vi "Main.vi"() -> ()   [LabVIEW 2016]
doc: "The myRIO Project template acquires acceleration data from the onboard accelerometer and displays the changes of acceleration values in a waveform chart."
uses:
  <vilib>/myRIO/Instrument Drivers/Onboard IO/PWM/typedefs/PWM Reference.ctl
  <vilib>/myRIO/Common/Instrument Driver Framework/Utilities/typedefs/myRIO Generic Hardware Reference.ctl
  <vilib>/myRIO/Common/Instrument Driver Framework/Utilities/typedefs/Hardware Version Enum.ctl
  <vilib>/myRIO/Common/Instrument Driver Framework/Utilities/typedefs/myRIO v1.0 Reference.ctl
  <vilib>/myRIO/Common/Instrument Driver Framework/Utilities/typedefs/Generic FPGA Reference.ctl
  <vilib>/myRIO/Common/Instrument Driver Framework/myRIO v1.0/PWM/typedefs/PWM Channels Enum.ctl
  <vilib>/myRIO/Instrument Drivers/Onboard IO/PWM/typedefs/PWM Configuration.ctl
  <vilib>/userdefined/High Color/nirio_resource_hc.ctl
  <vilib>/myRIO/Common/Instrument Driver Framework/myRIO v1.0/PWM/vis/myRIO v1.1 Open PWM.vi
  <vilib>/myRIO/Common/Instrument Driver Framework/Utilities/vis/Validate Channels.vi
  <vilib>/myRIO/Common/Instrument Driver Framework/myRIO v1.0/PWM/vis/myRIO v1.0 Reserve PWM.vi
  <vilib>/myRIO/Common/Instrument Driver Framework/myRIO v1.0/UART/vis/myRIO v1.0 Close UART.vi
  <vilib>/myRIO/Common/Instrument Driver Framework/myRIO v1.0/PWM/vis/myRIO v1.0 Build MUX Configuration PWM.vi
  <vilib>/myRIO/Common/Instrument Driver Framework/myRIO v1.0/Resource Manager/vis/myRIO v1.0 Reserve Channel List.vi
  <vilib>/myRIO/Common/Instrument Driver Framework/myRIO v1.0/Resource Manager/vis/myRIO v1.0 Create Configuration List.vi
  <vilib>/myRIO/Common/Instrument Driver Framework/myRIO v1.0/Resource Manager/vis/myRIO v1.0 Reserve Channel.vi
  <vilib>/myRIO/Common/Instrument Driver Framework/myRIO v1.0/Resource Manager/vis/myRIO v1.0 Unreserve Channel.vi
  <vilib>/myRIO/Common/Instrument Driver Framework/myRIO v1.0/Resource Manager/vis/myRIO v1.0 Build Mutex Name.vi
  <vilib>/Utility/VariantDataType/GetNumericInfo.vi
  <vilib>/Utility/error.llb/Error Cluster From Error Code.vi
  <vilib>/myRIO/Common/Instrument Driver Framework/myRIO v1.0/myRIO v1.1 Open.vi
  <vilib>/myRIO/Common/Instrument Driver Framework/Utilities/vis/IO Manager.vi
  <vilib>/myRIO/Common/Instrument Driver Framework/Utilities/vis/Configuration Manager.vi
  <vilib>/myRIO/Common/Instrument Driver Framework/myRIO v1.0/Resource Manager/vis/myRIO v1.0 Configure IO.vi
  <vilib>/myRIO/Common/Instrument Driver Framework/myRIO v1.0/myRIO v1.0 Close.vi
  <vilib>/addons/control/pid/pid.llb/PID (DBL).vi
  <vilib>/myRIO/Common/Instrument Driver Framework/myRIO v1.0/PWM/vis/myRIO v1.0 Write PWM.vi
  <vilib>/myRIO/Common/Instrument Driver Framework/Utilities/vis/FPGA Ref Manager.vi
  <vilib>/myRIO/Common/Instrument Driver Framework/myRIO v1.0/myRIO v1.0 Reset FPGA.vi
  <vilib>/myRIO/Common/Instrument Driver Framework/myRIO v1.0/IRQ/vis/myRIO v1.0 IRQ Info FGV.vi
  <vilib>/myRIO/Common/Instrument Driver Framework/myRIO v1.0/IRQ/vis/myRIO v1.0 Timer IRQ Info FGV.vi
  <vilib>/myRIO/Common/Instrument Driver Framework/myRIO v1.0/IRQ/vis/myRIO v1.0 ISR Agent.vi
  <vilib>/myRIO/Instrument Drivers/Onboard IO/PWM/vis/myRIO PWM Open.xnode
  <vilib>/myRIO/Instrument Drivers/Onboard IO/PWM/PWM.lvlib
  <vilib>/myRIO/Instrument Drivers/Utilities/Utilities.lvlib
  <vilib>/addons/control/pid/NI_PID_pid.lvlib
panel:
  out "output array":dbl[](array[numeric])
  in  "Stop Button":bool
  in  "y":dbl(knob) scale=0.0..1.0
  out "pwm motor":dbl
  in  "Frequenz Motor":dbl=200.0
  in  "stop 2":bool
  in  "PID gains":T1={"proportional gain (Kc)"=0.71, "integral time (Ti, min)"=2.0, "derivative time (Td, min)"=0.0015} {"derivative time (Td, min)" format="%.3f"; "integral time (Ti, min)" format="%.3f"; "proportional gain (Kc)" format="%.3f"}
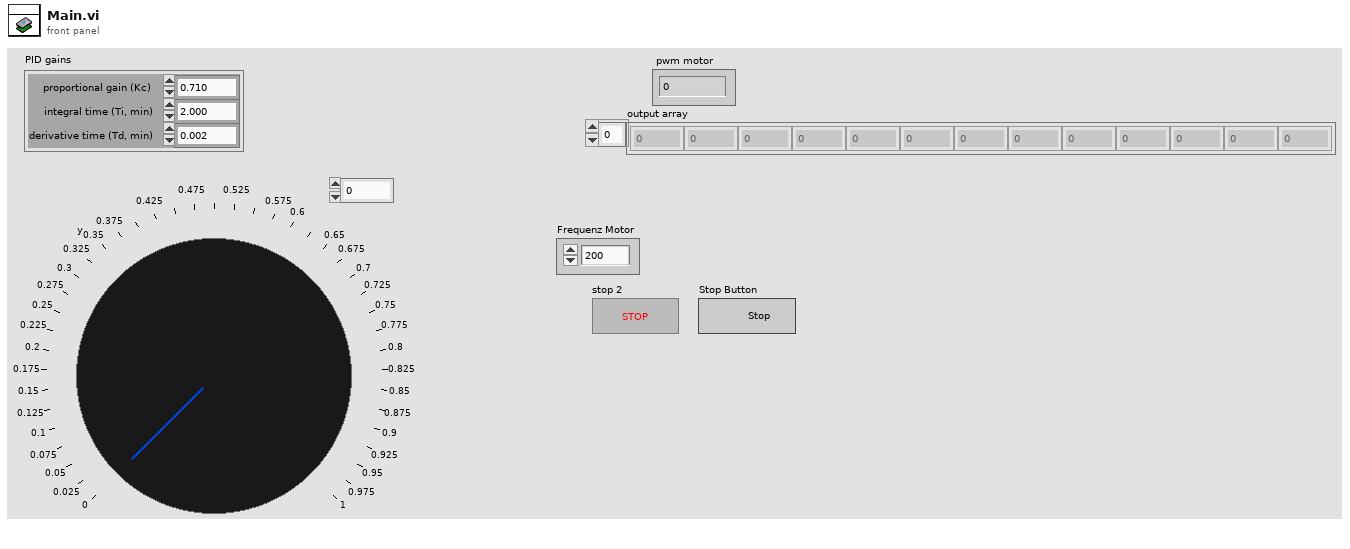
[diagram p1: front panel]
types:
  T1 = cluster{"proportional gain (Kc)":dbl, "integral time (Ti, min)":dbl, "derivative time (Td, min)":dbl}
  T2 = typedef "PWM.lvlib/PWM Reference.ctl" = cluster{"myRIO Reference":T3, "PWM Channels Enum":T7, "PWM Configuration":T8}
  T3 = typedef "myRIO Generic Hardware Reference.ctl" = cluster{"myRIO Model":T4, "myRIO Hardware Reference":T5}
  T4 = typedef "Hardware Version Enum.ctl" = enum16{"Unknown", "myRIO-1900", "myRIO-1950", "roboRIO", "NI ELVIS RIO CM"}
  T5 = typedef "myRIO v1.0 Reference.ctl" = cluster{"Generic FPGA Reference":T6, "Allow multiple opens":bool}
  T6 = typedef "Generic FPGA Reference.ctl" = refnum<k20>
  T7 = typedef "PWM Channels Enum.ctl" = enum16{"Not Connected", "C/PWM0", "C/PWM1", "A/PWM0", "A/PWM1", "A/PWM2", "B/PWM0", "B/PWM1", "B/PWM2", "PWM/PWM0", "PWM/PWM1", "PWM/PWM2", "PWM/PWM3", "PWM/PWM4", "PWM/PWM5", "PWM/PWM6", "PWM/PWM7", "PWM/PWM8", "PWM/PWM9"}
  T8 = typedef "PWM.lvlib/PWM Configuration.ctl" = cluster{"Frequency":dbl, "Duty Cycle":dbl}
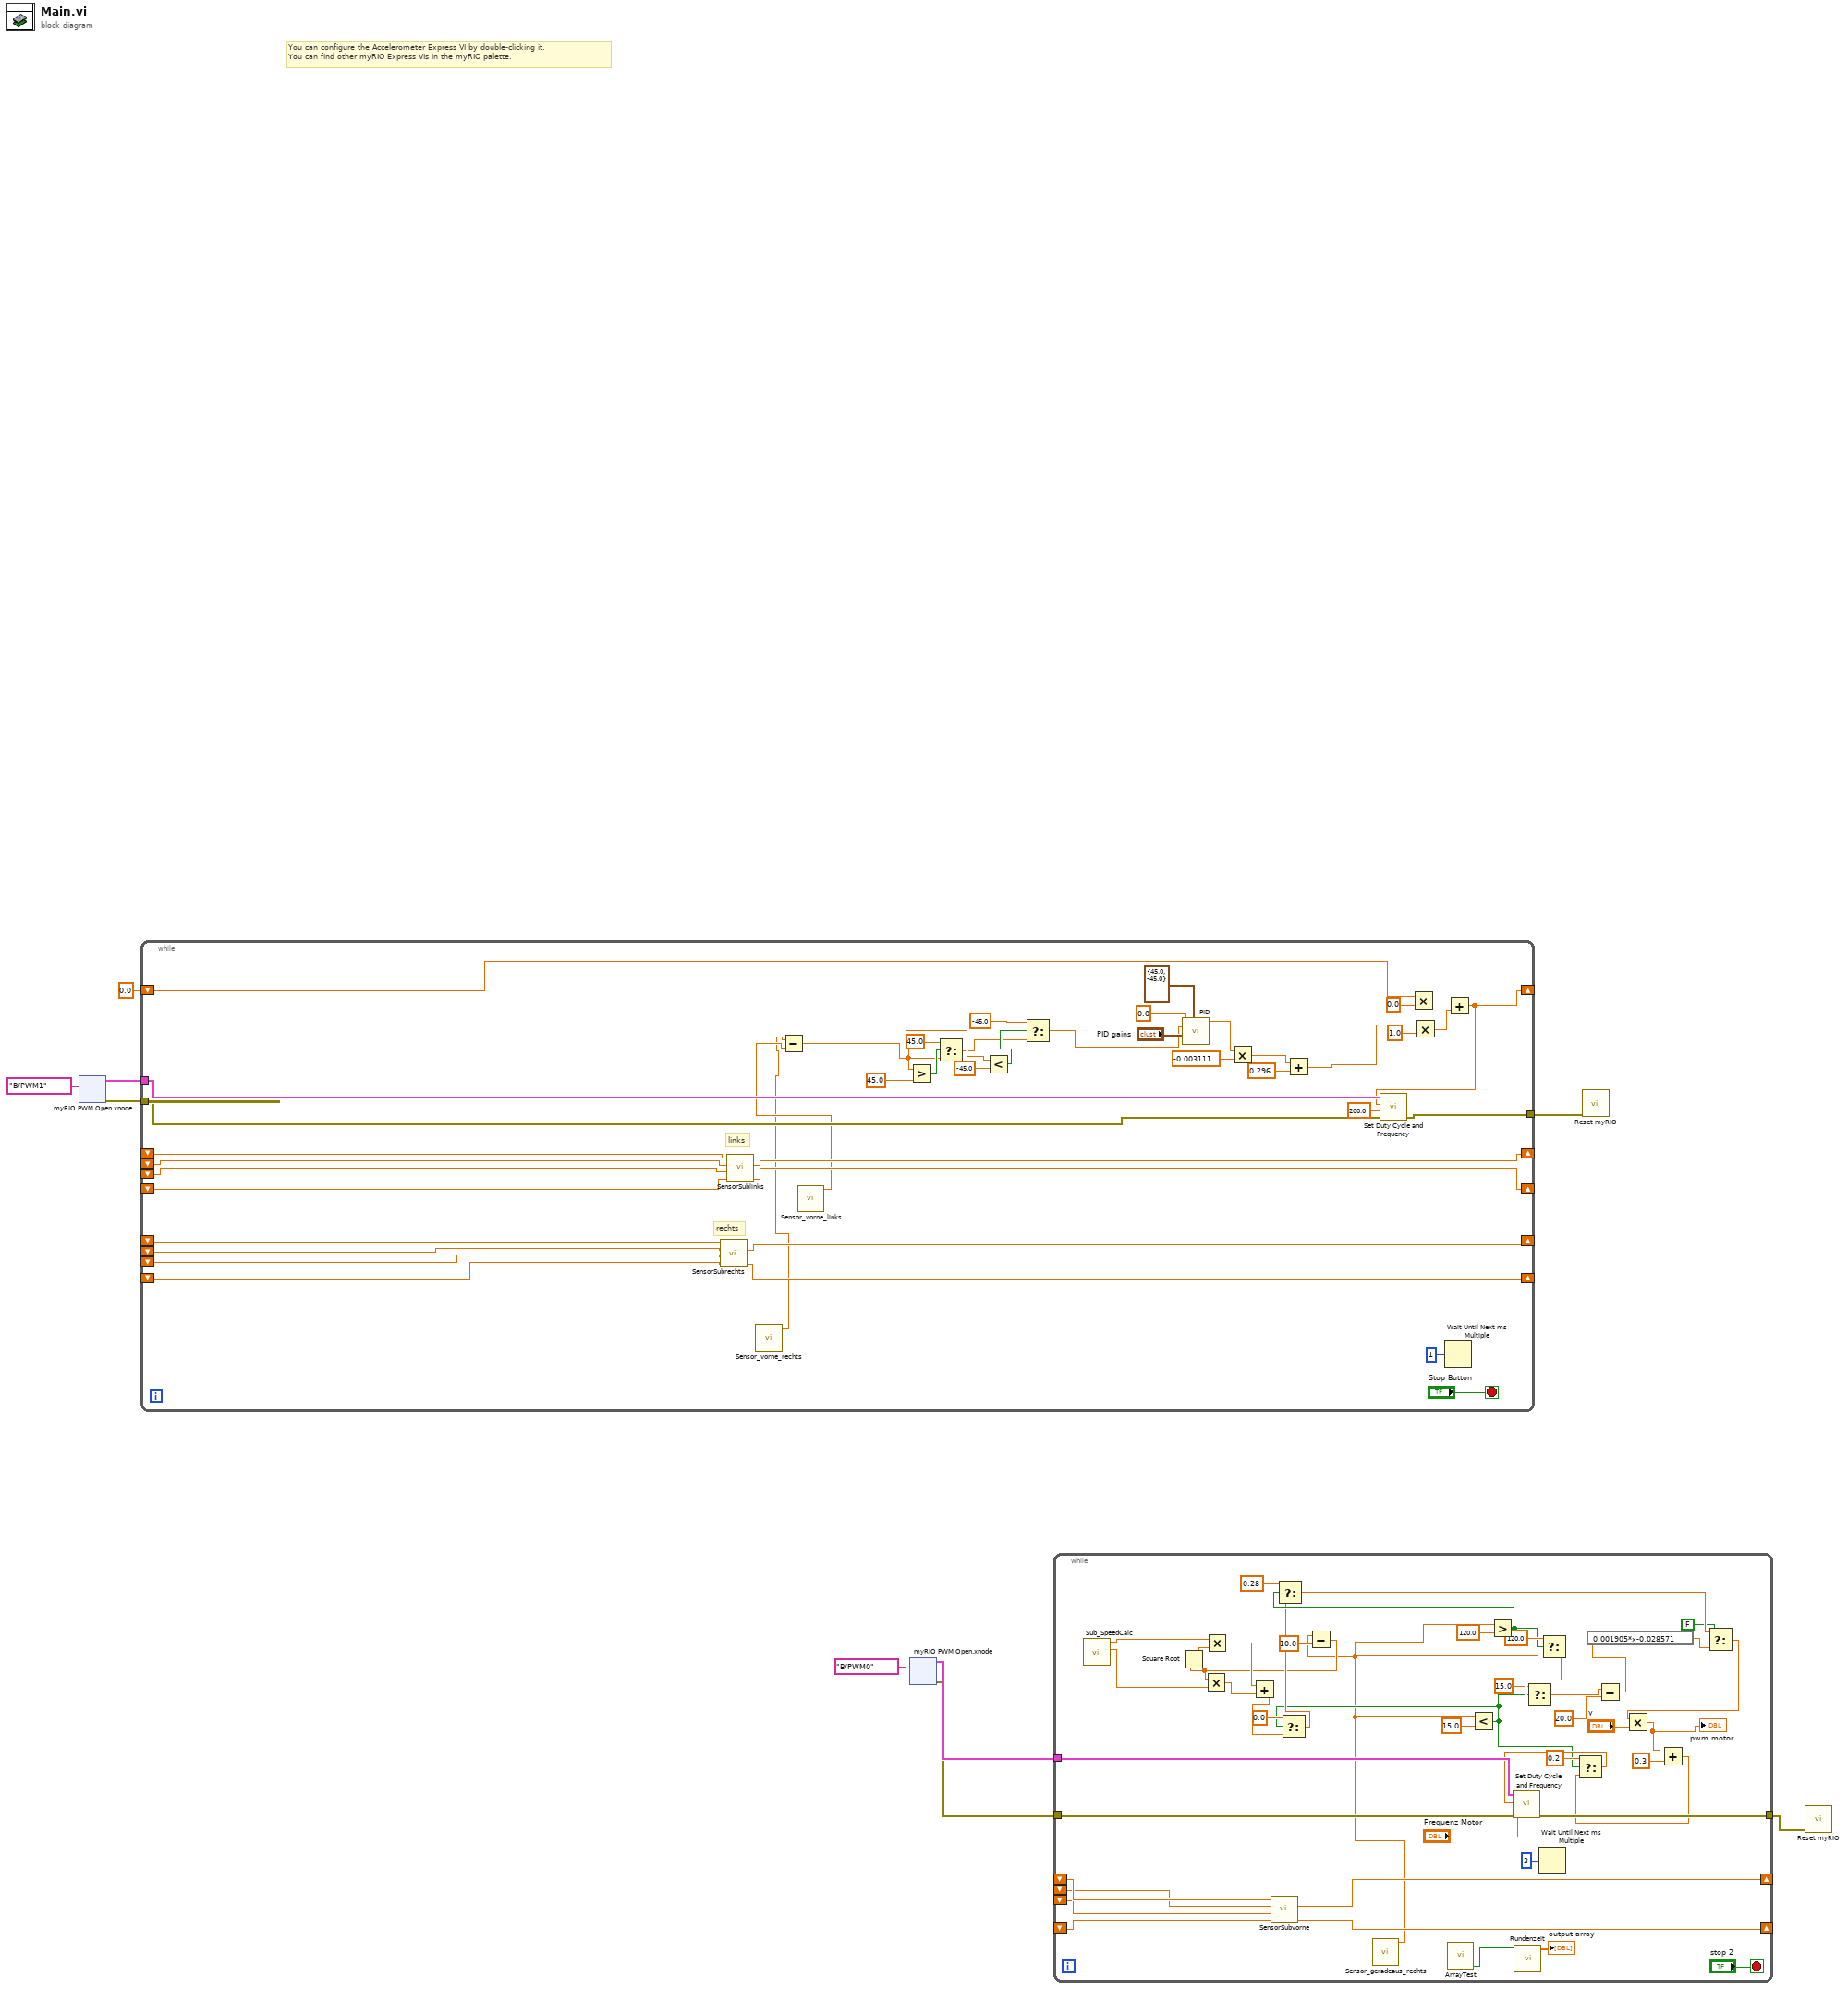
[diagram p0: block diagram]
diagram:
  # "You can configure the Accelerometer Express VI by double-clicking it.\nYou can find other myRIO Express VIs in the myRIO palette."
  n1 = xnode "myRIO PWM Open.xnode"("Channel Name"=tag "B/PWM1") -> ("error out"=w8:errorcluster, "PWM Ref Out"=w7:T2)  [unwired: 2 in]
  n2 = while {
    tunnel: w8 -> [w50]
    tunnel: w7 -> [w52]
    tunnel: [w51] -> w6
    shift-right: [w30] -> _
    shift-left: _ -> [w31]
    shift-right: [w29] -> _
    shift-left: _ -> [w34]
    shift-left: _ -> [w33]
    shift-left: _ -> [w32]
    shift-right: [w42] -> _
    shift-left: 0.0 -> [w45]
    shift-right: [w23] -> _
    shift-left: _ -> [w28]
    shift-left: _ -> [w27]
    shift-left: _ -> [w26]
    shift-right: [w24] -> _
    shift-left: _ -> [w25]
    stop <- "Stop Button" stop-if-true
    # "links"
    # "rechts"
    n3 = call "SensorSubrechts.vi"("Tiefpass in"=w25, "element 3"=w26, "element 2"=w27, "element"=w28) -> ("Tiefpass out"=w24:dbl, "Ausgabe IR"=w23:dbl)  [unwired: 5 in, 1 out]
    n4 = call "SensorSublinks.vi"("Tiefpass in"=w31, "element 3"=w32, "element 2"=w33, "element"=w34) -> ("Tiefpass out"=w30:dbl, "Ausgabe IR"=w29:dbl)  [unwired: 5 in, 1 out]
    n5 = call "Sensor_vorne_rechts.vi"() -> ("Abstand in cm"=w10:dbl)  [unwired: 11 in]
    n6 = call "Sensor_vorne_links.vi"() -> ("Abstand in cm"=w11:dbl)  [unwired: 11 in]
    n7 = Subtract(x=w10, y=w11) -> (x-y=w15:dbl)
    n8 = Greater?(x=w15, y=45.0) -> (0:w21:bool)
    n9 = Select(t=45.0, s=w21, f=w15) -> (s? t:f=w14:dbl)
    n10 = Less?(x=w15, y=-45.0) -> (x < y?=w16:bool)
    n11 = Select(t=-45.0, s=w16, f=w14) -> (s? t:f=w13:dbl)
    n12 = call-poly <vilib>:"PID.vi"("output range"=cluster{"output high":dbl, "output low":dbl} {"output high"=45.0, "output low"=-45.0}, "PID gains"="PID gains", "process variable"=w13, "setpoint"=0.0) -> ("output"=w22:dbl)  [unwired: 6 in, 1 out]
    n13 = Multiply(x=w22, y=-0.003111) -> (x*y=w38:dbl)
    n14 = Add(x=w38, y=0.296) -> (x+y=w36:dbl)
    n15 = Multiply(x=w45, y=0.0) -> (x*y=w44:dbl)
    n16 = Multiply(x=w36, y=1.0) -> (x*y=w43:dbl)
    n17 = Wait Until Next ms Multiple(millisecond multiple=u32 1) -> ()  [unwired: 1 out]
    n18 = Add(x=w44, y=w43) -> (x+y=w42:dbl)
    n19 = call <vilib>:"Set Duty Cycle and Frequency.vi"("error in (no error)"=w50, "Frequency [Hz]"=200.0 ("y"), "Duty Cycle"=w42, "PWM Ref In"=w52) -> ("error out"=w51:errorcluster)  [unwired: 5 in, 1 out]
  }
  n20 = xnode "myRIO PWM Open.xnode"("Channel Name"=tag "B/PWM0") -> ("error out"=w2:errorcluster, "PWM Ref Out"=w3:T2)  [unwired: 2 in]
  n21 = while {
    tunnel: w3 -> [w97]
    tunnel: w2 -> [w96]
    tunnel: [w95] -> w1
    shift-right: [w91] -> _
    shift-left: _ -> [w92]
    shift-left: _ -> [w90]
    shift-left: _ -> [w89]
    shift-right: [w88] -> _
    shift-left: _ -> [w87]
    stop <- "stop 2" stop-if-true
    n22 = call "Sub_SpeedCalc.vi"() -> ("a"=w78:dbl, "b"=w77:dbl)  [unwired: 8 in]
    n23 = call "SensorSubvorne.vi"("Tiefpass in"=w87, "element 3"=w89, "element 2"=w90, "element"=w92) -> ("Tiefpass out"=w88:dbl, "Ausgabe IR"=w91:dbl)  [unwired: 5 in, 1 out]
    n24 = call "Sensor_geradeaus_rechts.vi"() -> ("Abstand in cm"=w55:dbl)  [unwired: 11 in]
    n25 = Subtract(x=w55, y=10.0) -> (x-y=w60:dbl)
    n26 = Square Root(x=w60) -> (sqrt(x)=w79:dbl)
    n27 = Multiply(x=w60, y=w77) -> (x*y=w75:dbl)
    n28 = Multiply(x=w78, y=w79) -> (x*y=w76:dbl)
    n29 = Add(x=w76, y=w75) -> (x+y=w62:dbl)
    n30 = call "ArrayTest.vi"() -> ("8 IR true"=w54:bool)  [unwired: 9 in, 1 out]
    n31 = Less?(x=w55, y=15.0) -> (x < y?=w56:bool)
    n32 = Select(t=0.0, s=w56, f=w62) -> (s? t:f=w71:dbl)
    n33 = Greater?(x=w55, y=120.0) -> (0:w74:bool)
    n34 = Select(t=0.28, s=w74, f=w71) -> (s? t:f=w68:dbl)
    n35 = call "Rundenzeit.vi"("8 IR true"=w54) -> ("output array"=→"output array":dbl[])  [unwired: 10 in]
    n36 = Wait Until Next ms Multiple(millisecond multiple=u32 3) -> ()  [unwired: 1 out]
    n37 = Select(t=120.0, s=w74, f=w55) -> (s? t:f=w84:dbl)
    n38 = Select(t=15.0, s=w56, f=w84) -> (s? t:f=w64:dbl)
    n39 = Subtract(x=w64, y=20.0) -> (x-y=w63:dbl)
    n40 = expression code="0.001905*x-0.028571"(w63) -> (w69:dbl)
    n41 = Select(t=w68, s=FALSE, f=w69) -> (s? t:f=w70:dbl)
    n42 = Multiply(x=w70, y="y") -> (x*y=w81:dbl)
    "pwm motor" <- w81
    n43 = Add(x=w81, y=0.3) -> (x+y=w59:dbl)
    n44 = Select(t=0.2, s=w56, f=w59) -> (s? t:f=w58:dbl)
    n45 = call <vilib>:"Set Duty Cycle and Frequency.vi"("error in (no error)"=w96, "Frequency [Hz]"="Frequenz Motor", "Duty Cycle"=w58, "PWM Ref In"=w97) -> ("error out"=w95:errorcluster)  [unwired: 5 in, 1 out]
  }
  n46 = call <vilib>:"Reset myRIO.vi"("error in (no error)"=w6) -> ()  [unwired: 10 in, 1 out]
  n47 = call <vilib>:"Reset myRIO.vi"("error in (no error)"=w1) -> ()  [unwired: 10 in, 1 out]
